vi "农业监测系统.vi"() -> ()   [LabVIEW 2013]
uses:
  <vilib>/Instr/_visa.llb/VISA Configure Serial Port (Instr).vi
panel:
  out "光照值":dbl
  out "光照计":dbl(slide) scale=0.0..30000.0
  in  "stop bits (10: 1 bit)":u16(ring)=10 caption="停止位（10: 1位）" items=["1.0"=10, "1.5"=15, "2.0"=20]
  in  "data bits (8)":u16=8 caption="数据比特(8)" min=5 max=8 step=1
  in  "baud rate (9600)":u32=9600 caption="波特率(9600)"
  in  "VISA resource name":refnum<visa-resource-name> caption="VISA资源名称"
  out "湿度值":dbl
  out "温度值":dbl
  out "湿度计":dbl(slide) scale=0.0..100.0
  out "温度计":dbl(slide) scale=0.0..100.0
  # "基于arduino的农业监控系统"
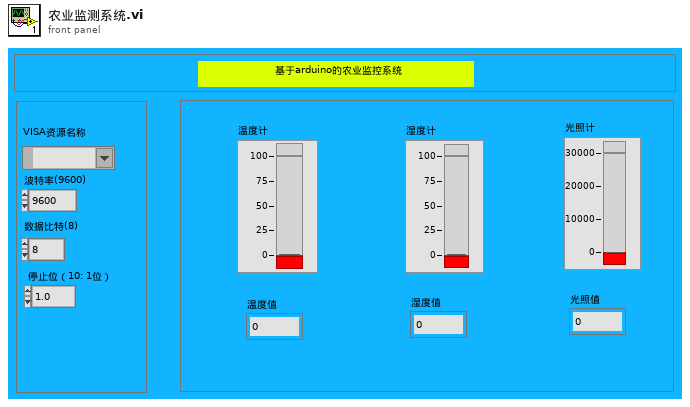
[diagram p1: front panel]
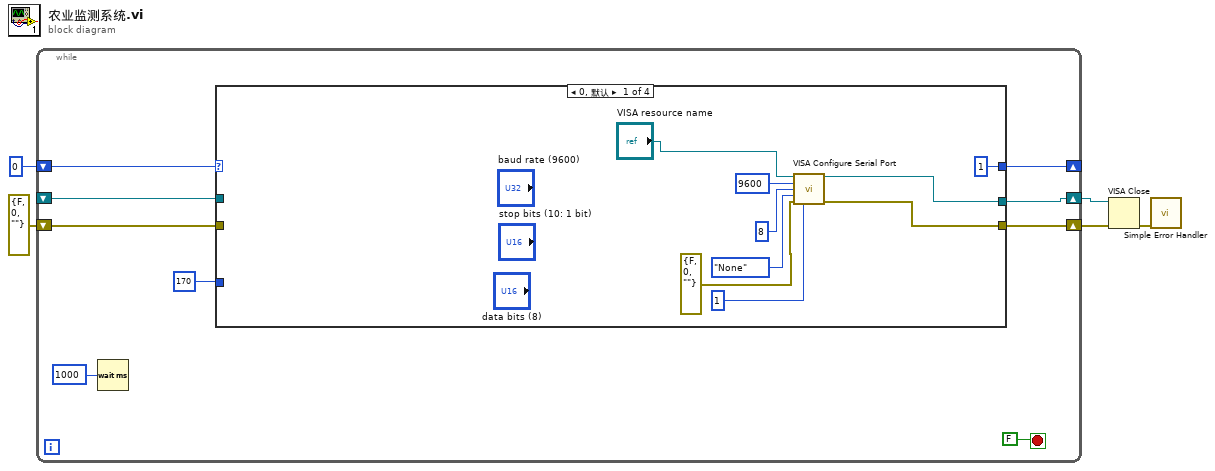
[diagram p0: block diagram]
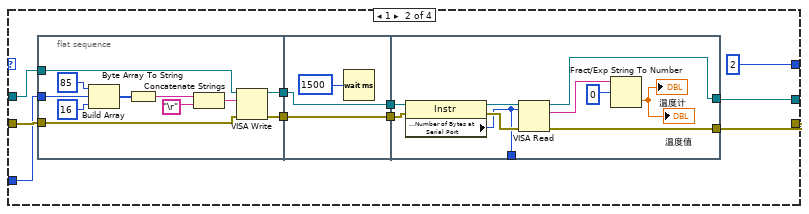
[diagram p2: hidden frame]
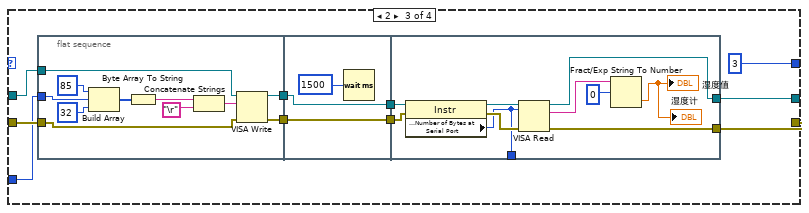
[diagram p3: hidden frame]
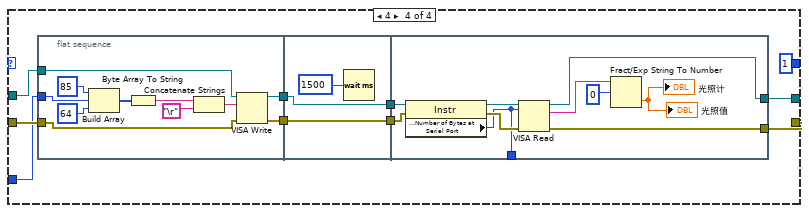
[diagram p4: hidden frame]
diagram:
  n1 = while {
    shift-right: [w14] -> w3
    shift-left: _ -> [w9]
    shift-right: [w13] -> w4
    shift-left: errorcluster {"status"=FALSE, "code"=0, "source"=""} ("error out") -> [w8]
    shift-right: [w12] -> _
    shift-left: 0 -> [w11]
    stop <- FALSE stop-if-true
    n2 = Wait (ms)(milliseconds to wait=u32 1000 ("等待时间（毫秒）")) -> ()  [unwired: 1 out]
    n3 = case shown="0, 默认" w11 {
      tunnel: [w18 w26 w60 w92] -> w14
      tunnel: [w20 w25 w59 w93] -> w13
      tunnel: [1 2 3 1] -> w12
      tunnel: w9 -> [_ w28 w62 w96]
      tunnel: w8 -> [_ w27 w61 w95]
      tunnel: 170 -> [_ w24 w58 w94]
      frame 0, Default {
        n4 = call-poly "VISA Configure Serial Port"("VISA resource name"="VISA resource name", "baud rate (9600)"=u32 9600, "data bits (8)"=u16 8, "parity (0:none)"=enum16{"None", "Odd", "Even", "Mark", "Space"}."None", "error in (no error)"=errorcluster {"status"=FALSE, "code"=0, "source"=""}, "stop bits (10: 1 bit)"=u32 1 ("Bytes at Port")) -> ("VISA resource name out"=w18:refnum<visa-resource-name>, "error out"=w20:errorcluster)  [unwired: 8 in]
      }
      frame 1 {
        n5 = flat-sequence {
          tunnel: [w38] -> w32
          tunnel: [w37] -> w31
          tunnel: w28 -> [w36]
          tunnel: w27 -> [w35]
          tunnel: w24 -> [w34]
          tunnel: w32 -> [w47]
          tunnel: w31 -> [w46]
          tunnel: [w47] -> w30
          tunnel: [w46] -> w29
          tunnel: w30 -> [w53]
          tunnel: w29 -> [w52]
          tunnel: [w51] -> w25
          tunnel: [w50] -> w26
          tunnel: [w49] -> _
          frame #0 {
            n6 = Build Array(85, w34, 16) -> (w43:i32[])
            n7 = Byte Array To String(unsigned byte array=w43) -> (string=w39:string)
            n8 = Concatenate Strings(w39, "\r") -> (w40:string)
            n9 = VISA Write(VISA resource name=w36, write buffer=w40, error in (no error)=w35) -> (VISA resource name out=w38:refnum<visa-resource-name>, error out=w37:errorcluster)  [unwired: 1 out]
          }
          frame #1 {
            n10 = Wait (ms)(milliseconds to wait=u32 1500 ("等待时间（毫秒）")) -> ()  [unwired: 1 out]
          }
          frame #2 {
            n11 = property class="Instr"(reference=w53, error in=w52) -> (reference out=w55:refnum<visa-resource-name>, error out=w54:errorcluster, "Serial Settings:Number of Bytes at Serial Port"=w49:u32)
            n12 = VISA Read(VISA resource name=w55, byte count=w49, error in (no error)=w54) -> (VISA resource name out=w50:refnum<visa-resource-name>, read buffer=w56:string, error out=w51:errorcluster)  [unwired: 1 out]
            n13 = Fract/Exp String To Number(string=w56, offset=0 ("偏移量")) -> (number=→"温度值" →"温度计":dbl)  [unwired: 2 in, 1 out]
          }
        }
      }
      frame 2 {
        n14 = flat-sequence {
          tunnel: [w72] -> w66
          tunnel: [w71] -> w65
          tunnel: w62 -> [w70]
          tunnel: w61 -> [w69]
          tunnel: w58 -> [w68]
          tunnel: w66 -> [w81]
          tunnel: w65 -> [w80]
          tunnel: [w81] -> w64
          tunnel: [w80] -> w63
          tunnel: w64 -> [w87]
          tunnel: w63 -> [w86]
          tunnel: [w85] -> w59
          tunnel: [w84] -> w60
          tunnel: [w83] -> _
          frame #0 {
            n15 = Build Array(85, w68, 32) -> (w77:i32[])
            n16 = Byte Array To String(unsigned byte array=w77) -> (string=w73:string)
            n17 = Concatenate Strings(w73, "\r") -> (w74:string)
            n18 = VISA Write(VISA resource name=w70, write buffer=w74, error in (no error)=w69) -> (VISA resource name out=w72:refnum<visa-resource-name>, error out=w71:errorcluster)  [unwired: 1 out]
          }
          frame #1 {
            n19 = Wait (ms)(milliseconds to wait=u32 1500 ("等待时间（毫秒）")) -> ()  [unwired: 1 out]
          }
          frame #2 {
            n20 = property class="Instr"(reference=w87, error in=w86) -> (reference out=w89:refnum<visa-resource-name>, error out=w88:errorcluster, "Serial Settings:Number of Bytes at Serial Port"=w83:u32)
            n21 = VISA Read(VISA resource name=w89, byte count=w83, error in (no error)=w88) -> (VISA resource name out=w84:refnum<visa-resource-name>, read buffer=w90:string, error out=w85:errorcluster)  [unwired: 1 out]
            n22 = Fract/Exp String To Number(string=w90, offset=0 ("偏移量")) -> (number=→"湿度值" →"湿度计":dbl)  [unwired: 2 in, 1 out]
          }
        }
      }
      frame 4 {
        n23 = flat-sequence {
          tunnel: [w106] -> w100
          tunnel: [w105] -> w99
          tunnel: w96 -> [w104]
          tunnel: w95 -> [w103]
          tunnel: w94 -> [w102]
          tunnel: w100 -> [w115]
          tunnel: w99 -> [w114]
          tunnel: [w115] -> w98
          tunnel: [w114] -> w97
          tunnel: w98 -> [w121]
          tunnel: w97 -> [w120]
          tunnel: [w119] -> w93
          tunnel: [w118] -> w92
          tunnel: [w117] -> _
          frame #0 {
            n24 = Build Array(85, w102, 64) -> (w111:i32[])
            n25 = Byte Array To String(unsigned byte array=w111) -> (string=w107:string)
            n26 = Concatenate Strings(w107, "\r") -> (w108:string)
            n27 = VISA Write(VISA resource name=w104, write buffer=w108, error in (no error)=w103) -> (VISA resource name out=w106:refnum<visa-resource-name>, error out=w105:errorcluster)  [unwired: 1 out]
          }
          frame #1 {
            n28 = Wait (ms)(milliseconds to wait=u32 1500 ("等待时间（毫秒）")) -> ()  [unwired: 1 out]
          }
          frame #2 {
            n29 = property class="Instr"(reference=w121, error in=w120) -> (reference out=w123:refnum<visa-resource-name>, error out=w122:errorcluster, "Serial Settings:Number of Bytes at Serial Port"=w117:u32)
            n30 = VISA Read(VISA resource name=w123, byte count=w117, error in (no error)=w122) -> (VISA resource name out=w118:refnum<visa-resource-name>, read buffer=w124:string, error out=w119:errorcluster)  [unwired: 1 out]
            n31 = Fract/Exp String To Number(string=w124, offset=0 ("偏移量")) -> (number=→"光照计" →"光照值":dbl)  [unwired: 2 in, 1 out]
          }
        }
      }
    }
  }
  n32 = VISA Close(VISA resource name=w3, error in (no error)=w4) -> (error out=w2:errorcluster)
  n33 = call <vilib>:"Simple Error Handler.vi"("error in (no error)"=w2) -> ()  [unwired: 4 in, 5 out]
